vi "AMC Queue Registry.vi"(6 "Properties in":T1, 8 "error in (no error)":errorcluster, 9 "Message Queue in":T2, 10 "Index":i32, 11 "Method":T3) -> (0 "error out":errorcluster, 1 "Message Queue out":T2, 2 "Number of Queues":i32, 3 "All Queues":T2[](array[typedef]), 4 "Properties out":T1, 5 "All Properties":T1[](array[typedef]))   [LabVIEW 2011, in "ART2 Test Panel.lvlib" / "TLB_Dependencies.lvlib"]
doc: "This VI maintains the list of host connections."
uses:
  TLB_Dependencies.lvlib
  amc_QueueRegistryMethod.ctl
  amc_Message Queue.ctl
  amc_Message.ctl
  Users/rkidagan/Dropbox/Atheros/ART2/Development/ART2 Test Panel/ART2 Test Panel/Components/Dependencies.llb/Keyed Array.ctl
  amc_QueueRegistryProperties.ctl
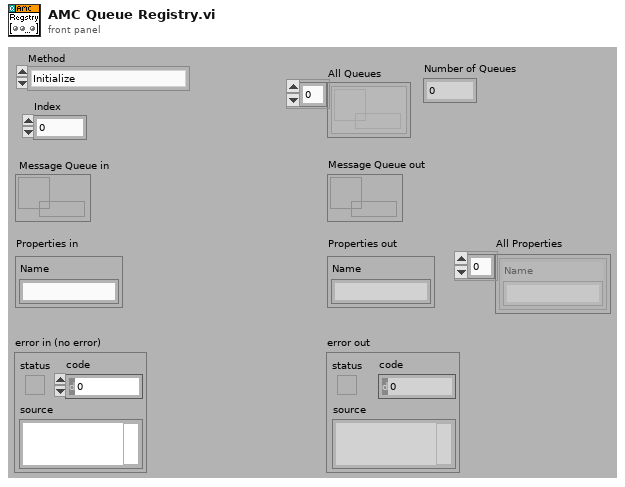
[diagram p1: front panel]
types:
  T1 = typedef "ART2 Test Panel.lvlib/TLB_Dependencies.lvlib/amc_QueueRegistryProperties.ctl" = cluster{"Name":string}
  T2 = typedef "ART2 Test Panel.lvlib/TLB_Dependencies.lvlib/amc_Message Queue.ctl" = refnum<queue>
  T3 = typedef "ART2 Test Panel.lvlib/TLB_Dependencies.lvlib/amc_QueueRegistryMethod.ctl" = enum16{"Initialize", "Add Queue", "Set Properties", "Get Queue by Index", "Get Queue by Name", "Remove Queue", "Remove All Queues"}
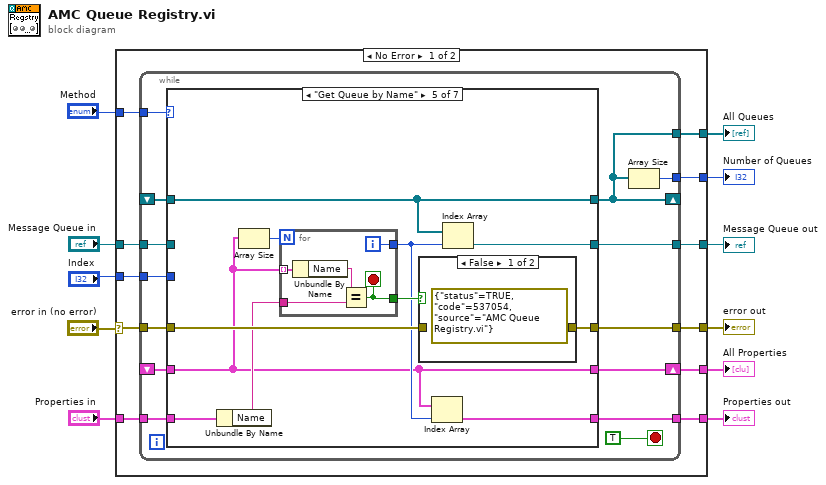
[diagram p0: block diagram]
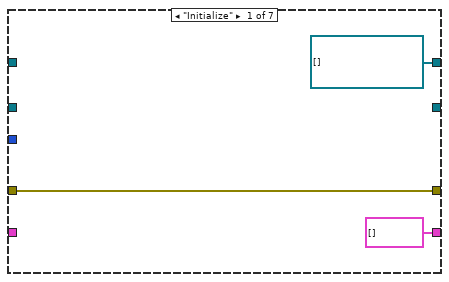
[diagram p2: hidden frame]
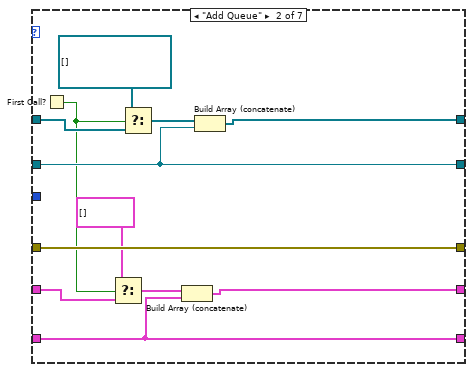
[diagram p3: hidden frame]
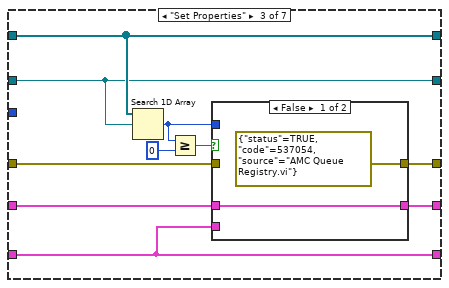
[diagram p4: hidden frame]
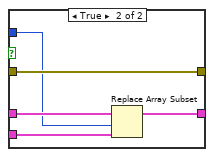
[diagram p5: hidden frame]
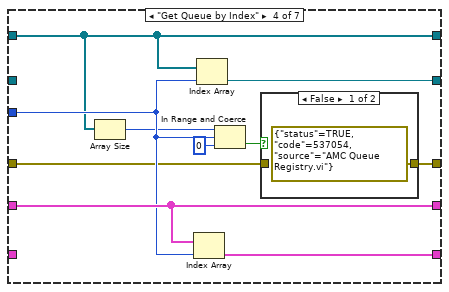
[diagram p6: hidden frame]
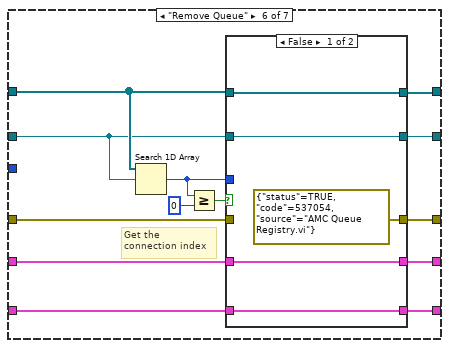
[diagram p9: hidden frame]
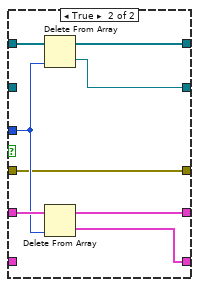
[diagram p10: hidden frame]
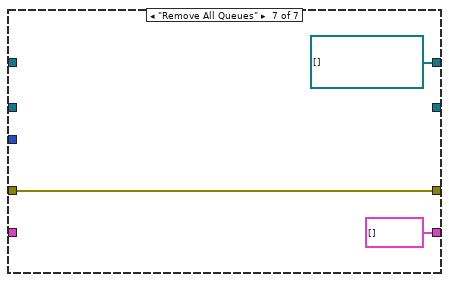
[diagram p11: hidden frame]
diagram:
  n1 = case shown="No Error" "error in (no error)" {
    selector: "error in (no error)" -> [w22 w129]
    tunnel: [w21 w129] -> w10
    tunnel: "Index" -> [w20 _]
    tunnel: "Method" -> [w19 _]
    tunnel: "Message Queue in" -> [w18 w128]
    tunnel: [w17 _] -> w6
    tunnel: [w16 _] -> w5
    tunnel: [w15 w128] -> w4
    tunnel: "Properties in" -> [w14 _]
    tunnel: [w13 _] -> w2
    tunnel: [w12 _] -> w1
    frame No Error {
      n2 = while {
        shift-right: [w28] -> _
        shift-left: _ -> [w35]
        tunnel: w22 -> [w34]
        tunnel: [w33] -> w21
        tunnel: w20 -> [w32]
        tunnel: w19 -> [w31]
        tunnel: w18 -> [w30]
        tunnel: [w29] -> w17
        tunnel: [w28] -> w16
        tunnel: [w27] -> w15
        shift-right: [w24] -> w13
        shift-left: _ -> [w26]
        tunnel: w14 -> [w25]
        tunnel: [w23] -> w12
        stop <- TRUE stop-if-true
        n3 = case shown="\"Get Queue by Name\"" w31 {
          tunnel: w35 -> [_ w46 w60 w74 w89 w111 _]
          tunnel: w30 -> [_ w50 w59 _ _ w103 _]
          tunnel: [T2[] [] w51 w60 w74 w89 w107 T2[] []] -> w28
          tunnel: [_ w50 w59 w78 w91 w106 _] -> w27
          tunnel: [w39 w49 w56 w69 w87 w105 w127] -> w33
          tunnel: w34 -> [w39 w49 w57 w72 w88 w104 w127]
          tunnel: w32 -> [_ _ _ w75 _ _ _]
          tunnel: w26 -> [_ w41 w55 w77 w81 w102 _]
          tunnel: w25 -> [_ w47 w52 _ w86 w99 _]
          tunnel: [T1[] [] w48 w53 w77 w81 w101 T1[] []] -> w24
          tunnel: [_ w47 w52 w76 w90 w100 _] -> w23
          frame "Initialize" {
          }
          frame "Add Queue" {
            n4 = First Call?() -> (First Call?: T/F=w42:bool)
            n5 = Select(t=T1[] [], s=w42, f=w41) -> (s? t:f=w43:T1[])
            n6 = Select(t=T2[] [], s=w42, f=w46) -> (s? t:f=w45:T2[])
            n7 = Build Array (concatenate)(w43, w47) -> (w48:T1[])
            n8 = Build Array (concatenate)(w45, w50) -> (w51:T2[])
          }
          frame "Set Properties" {
            n9 = Search 1D Array(1D array=w60, element=w59) -> (index of element=w54:i32)  [unwired: 1 out]
            n10 = Greater Or Equal?(x=w54, y=0) -> (x >= y?=w58:bool)
            n11 = case shown="False" w58 {
              tunnel: w57 -> [_ w68]
              tunnel: [errorcluster {"status"=TRUE, "code"=537054, "source"="AMC Queue Registry.vi"} ("error IO") w68] -> w56
              tunnel: w55 -> [w63 w67]
              tunnel: w54 -> [_ w66]
              tunnel: w52 -> [_ w65]
              tunnel: [w63 w64] -> w53
              frame False {
              }
              frame True {
                n12 = Replace Array Subset(array=w67, new element=w65, index=w66) -> (w64:T1[])
              }
            }
          }
          frame "Get Queue by Index" {
            n13 = Array Size(array=w74) -> (size(s)=w73:i32)
            n14 = Index Array(array=w77, index=w75) -> (element=w76:T1)
            n15 = Index Array(array=w74, index=w75) -> (element=w78:T2)
            n16 = In Range and Coerce(upper limit=w73, x=w75, lower limit=0) -> (In Range?=w71:bool)  [unwired: 1 out]
            n17 = case shown="False" w71 {
              tunnel: w72 -> [_ w80]
              tunnel: [errorcluster {"status"=TRUE, "code"=537054, "source"="AMC Queue Registry.vi"} ("error IO") w80] -> w69
              frame False {
              }
              frame True {
              }
            }
          }
          frame "Get Queue by Name" {
            n18 = Unbundle By Name(w86) -> ("Name"=w84:string)
            n19 = Array Size(array=w81) -> (size(s)=w85:i32)
            n20 = for {
              N: w85 -> [_]
              tunnel: w81 -> [w96] mode=indexing
              tunnel: w84 -> [w94]
              tunnel: [w93] -> w83
              tunnel: [w92] -> w82
              i -> [w92]
              stop <- w93 stop-if-true
              n21 = Unbundle By Name(w96) -> ("Name"=w95:string)
              n22 = Equal?(x=w95, y=w94) -> (x = y?=w93:bool)
            }
            n23 = case shown="False" w83 {
              tunnel: w88 -> [_ w98]
              tunnel: [errorcluster {"status"=TRUE, "code"=537054, "source"="AMC Queue Registry.vi"} ("error IO") w98] -> w87
              frame False {
              }
              frame True {
              }
            }
            n24 = Index Array(array=w81, index=w82) -> (element=w90:T1)
            n25 = Index Array(array=w89, index=w82) -> (element=w91:T2)
          }
          frame "Remove Queue" {
            # "Get the \nconnection index"
            n26 = Search 1D Array(1D array=w111, element=w103) -> (index of element=w110:i32)  [unwired: 1 out]
            n27 = Greater Or Equal?(x=w110, y=0) -> (x >= y?=w108:bool)
            n28 = case shown="False" w108 {
              tunnel: w111 -> [w116 w123]
              tunnel: w110 -> [_ w120]
              tunnel: [w116 w124] -> w107
              tunnel: [w115 w118] -> w106
              tunnel: [errorcluster {"status"=TRUE, "code"=537054, "source"="AMC Queue Registry.vi"} ("error IO") w117] -> w105
              tunnel: w104 -> [_ w117]
              tunnel: w103 -> [w115 _]
              tunnel: w102 -> [w114 w122]
              tunnel: [w114 w121] -> w101
              tunnel: [w113 w119] -> w100
              tunnel: w99 -> [w113 _]
              frame False {
              }
              frame True {
                n29 = Delete From Array(array=w123, index=w120) -> (deleted portion=w118:T2, array with subset deleted=w124:T2[])  [unwired: 1 in]
                n30 = Delete From Array(array=w122, index=w120) -> (deleted portion=w119:T1, array with subset deleted=w121:T1[])  [unwired: 1 in]
              }
            }
          }
          frame "Remove All Queues" {
          }
        }
        n31 = Array Size(array=w28) -> (size(s)=w29:i32)
      }
    }
    frame Error {
    }
  }
  "error out" <- w10
  "Number of Queues" <- w6
  "All Queues" <- w5
  "Message Queue out" <- w4
  "All Properties" <- w2
  "Properties out" <- w1
